vi "SmoothTriangleWaveform.vi"(0 "error in":errorcluster caption="entrée d'erreur", 2 "Direction":enum16{"rising", "falling"}(ring), 5 "Offset":dbl[unit] min=0.0 max=1.0 step=0.01 format="%.2f", 6 "Stiffness":dbl=0.95 min=0.0 max=1.0 step=0.01 format="%.2f", 7 "Speed":dbl[unit]=10.0 format="%.2f", 9 "Linear Amplitude":dbl[unit]=8.0 format="%.2f", 10 "Delay":dbl[unit] format="%.2f") -> (3 "error out":errorcluster caption="sortie d'erreur", 8 "Smooth Triangle Waveform":waveform(dbl)(graph)={"t0"=timestamp(0 s since 1904-01-01), "dt"=0.00030517578125, "Y"=array[4096 elements]})   [LabVIEW 2009]
doc: "This VI generates a smooth triangle waveform with a leading delay.\n---------------------------------------------------------------------------------\nDelay: Delay requested between the linear part of the triangle and the begining of the waveform.\nSpeed: Speed of the linear part of the triangle.\nAmplitude: Amplitude of the triangular waveform (achieved only for a stifness=1).\nOffset: Offset to the traingular waveform.\nStiffness: Stiffness of the triangular waveform.\n (Stiffness=1) <=> (triangular waveform)\n (Stiffness=0) <=> (cosine waveform)\nDirection: Either rising or falling.\n---------------------------------------------------------------------------------\nThis VI was adapted\nby Julien WOILLEZ in May 2003\nfrom Cyril RUILIER March 1999 code"
uses:
  <vilib>/Analysis/NI_AALBase.lvlib
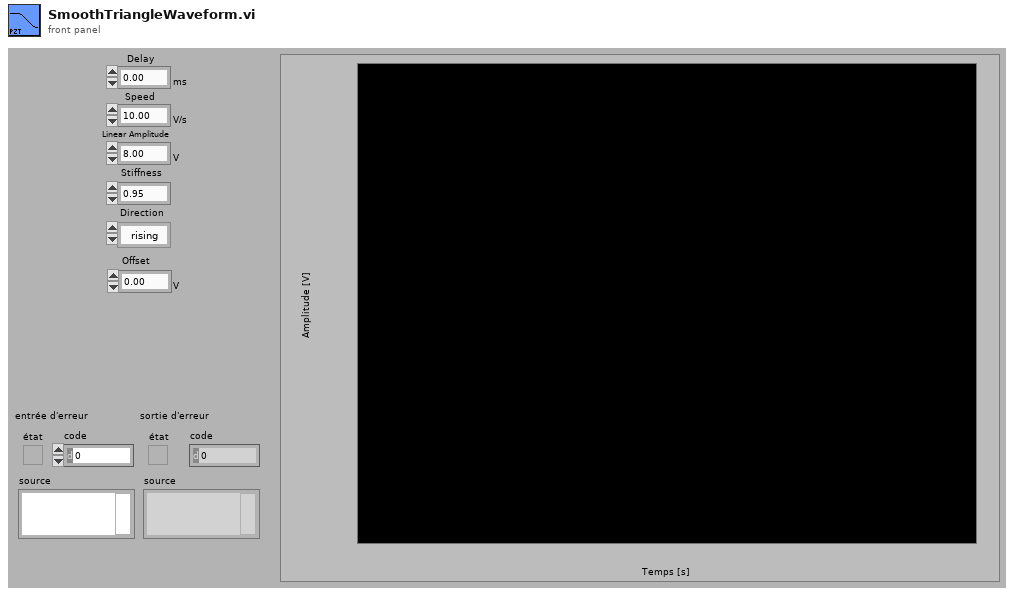
[diagram p1: front panel]
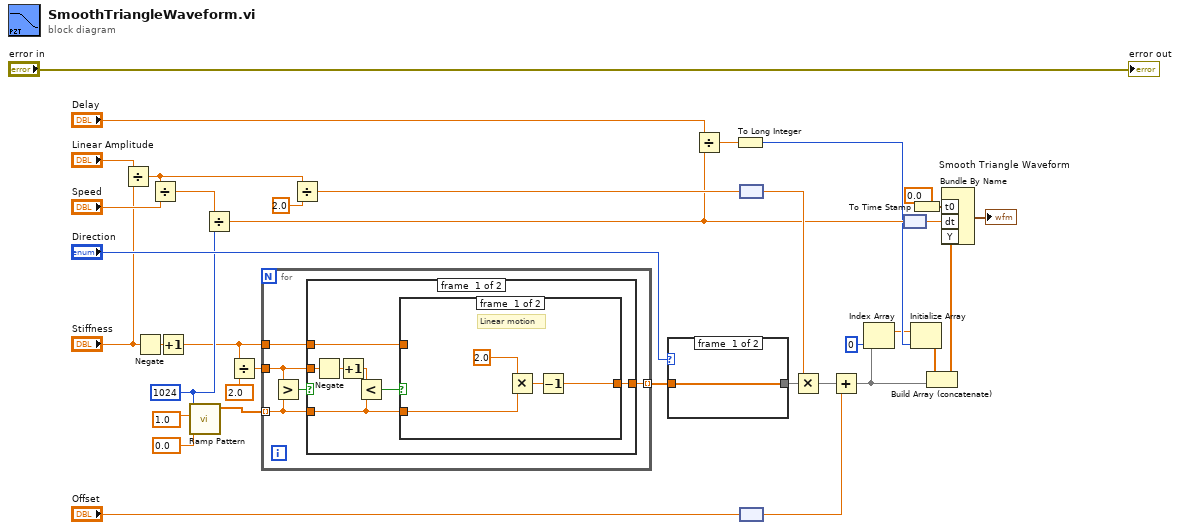
[diagram p0: block diagram]
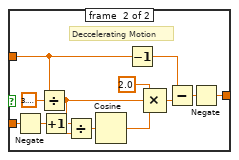
[diagram p2: hidden frame]
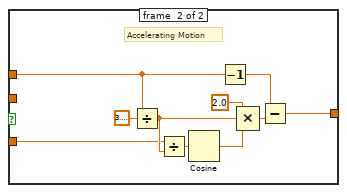
[diagram p3: hidden frame]
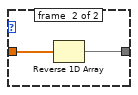
[diagram p4: hidden frame]
diagram:
  w29 = 1024 ("samples")
  n1 = Divide(x="Linear Amplitude", y="Stiffness") -> (x/y=w18:dbl[unit])
  n2 = Negate(x="Stiffness") -> (-x=w31:dbl)
  n3 = Divide(x=w18, y="Speed") -> (x/y=w14:dbl[unit])
  n4 = Increment(x=w31) -> (x+1=w15:dbl)
  n5 = call <vilib>:"Ramp Pattern.vi"("start"=0.0, "end"=1.0, "samples"=w29) -> ("Ramp Pattern"=w28:dbl[])  [unwired: 7 in, 1 out]
  n6 = Divide(x=w14, y=w29) -> (x/y=w12:dbl[unit])
  n7 = Divide(x=w15, y=2.0) -> (x/y=w27:dbl)
  n8 = for {
    tunnel: w28 -> [w39] mode=indexing
    tunnel: w27 -> [w41]
    tunnel: [w38] -> w25 mode=indexing
    tunnel: w15 -> [w37]
    n9 = Greater?(x=w41, y=w39) -> (0:w40:bool)
    n10 = case shown="True" w40 {
      tunnel: w39 -> [w47 w67]
      tunnel: [w48 w66] -> w38
      tunnel: w37 -> [w42 w68]
      tunnel: w41 -> [w46 _]
      frame #0 {
        n11 = Negate(x=w46) -> (-x=w45:dbl)
        n12 = Increment(x=w45) -> (x+1=w44:dbl)
        n13 = Less?(x=w44, y=w47) -> (x < y?=w43:bool)
        n14 = case shown="True" w43 {
          tunnel: w47 -> [w50 w54]
          tunnel: [w51 w56] -> w48
          tunnel: w42 -> [_ w58]
          frame #0 {
            # "Linear motion"
            n15 = Multiply(x=2.0 ("valeur"), y=w50) -> (x*y=w52:dbl)
            n16 = Decrement(x=w52) -> (x-1=w51:dbl)
          }
          frame #1 {
            # "Deccelerating Motion"
            n17 = Negate(x=w54) -> (-x=w55:dbl)
            n18 = Divide(x=w58, y=3.141592653589793) -> (x/y=w60:dbl)
            n19 = Increment(x=w55) -> (x+1=w53:dbl)
            n20 = Divide(x=w53, y=w60) -> (x/y=w64:dbl)
            n21 = Cosine(x=w64) -> (cos(x)=w63:dbl)
            n22 = Decrement(x=w58) -> (x-1=w62:dbl)
            n23 = Compound Arithmetic op=MULTIPLY(2.0 ("valeur"), w60, w63) -> (w61:dbl)
            n24 = Subtract(x=w62, y=w61) -> (x-y=w57:dbl)
            n25 = Negate(x=w57) -> (-x=w56:dbl)
          }
        }
      }
      frame #1 {
        # "Accelerating Motion"
        n26 = Divide(x=w68, y=3.141592653589793) -> (x/y=w74:dbl)
        n27 = Divide(x=w67, y=w74) -> (x/y=w70:dbl)
        n28 = Cosine(x=w70) -> (cos(x)=w71:dbl)
        n29 = Decrement(x=w68) -> (x-1=w72:dbl)
        n30 = Compound Arithmetic op=MULTIPLY(2.0 ("valeur"), w74, w71) -> (w73:dbl)
        n31 = Subtract(x=w72, y=w73) -> (x-y=w66:dbl)
      }
    }
  }
  n32 = Divide(x=w18, y=2.0) -> (x/y=w23:dbl[unit])
  n33 = case shown="\"falling\"" "Direction" {
    tunnel: w25 -> [w76 w77]
    tunnel: [w76 w78] -> w34
    frame #0 {
    }
    frame #1 {
      n34 = Reverse 1D Array(array=w77) -> (reversed array=w78:dbl[])
    }
  }
  n35 = Divide(x="Delay", y=w12) -> (x/y=w11:dbl)
  n36 = To Long Integer(number=w11) -> (32bit integer=w10:i32)
  n37 = node(w23) -> (w17:dbl)
  n38 = node("Offset") -> (w1:dbl)
  n39 = Multiply(x=w17, y=w34) -> (x*y=w4:dbl[])
  n40 = Add(x=w4, y=w1) -> (x+y=w3:dbl[])
  n41 = Index Array(array=w3, index=0 ("indice")) -> (element=w8:dbl)
  n42 = node(w12) -> (w22:dbl)
  n43 = Initialize Array(w8, w10) -> (w7:dbl[])
  n44 = To Time Stamp(1:0.0) -> (0:w5:timestamp)
  n45 = Build Array (concatenate)(w7, w3) -> (w6:dbl[])
  n46 = Bundle By Name("t0"=w5, "dt"=w22, "Y"=w6) -> (→"Smooth Triangle Waveform":waveform(dbl))  [unwired: 1 in]
  "error out" <- "error in"
